vi "get Error Code.vi"(8 "error in":errorcluster, 10 "errorNum":u32, 11 "cycloneHandle":u32) -> (0 "error out":errorcluster, 3 "function return":i32)   [LabVIEW 2021, in "CycloneControlSDK.lvlib"]
doc: "extern \"C\" int32_t _cdecl getErrorCode(uint32_t cycloneHandle, uint32_t errorNum);"
uses:
  CycloneControlSDK.lvlib
  CycloneControlSDK_64.dll
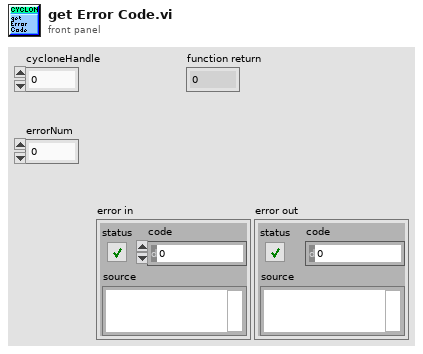
[diagram p1: front panel]
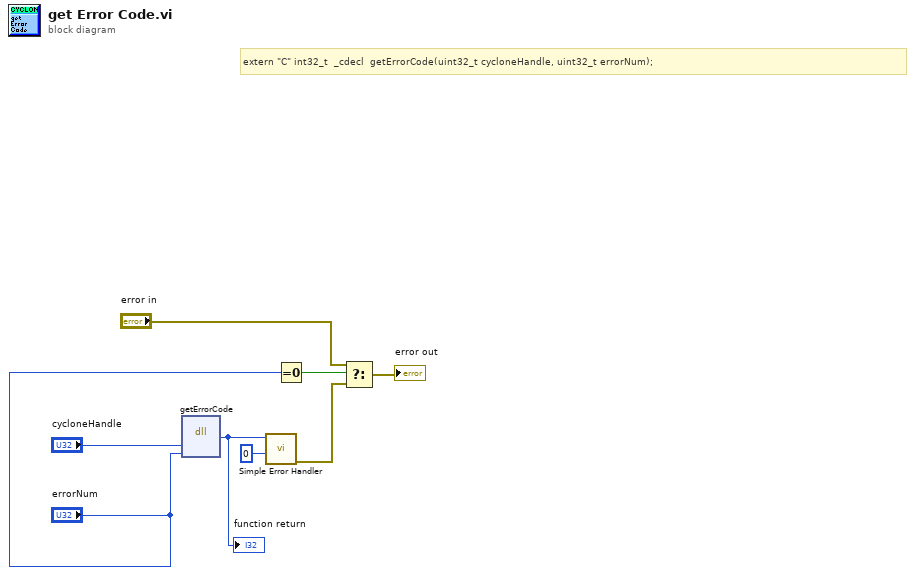
[diagram p0: block diagram]
diagram:
  # "extern \"C\" int32_t  _cdecl  getErrorCode(uint32_t cycloneHandle, uint32_t errorNum);"
  n1 = dll-call lib="C:/PEMicro/cyclone/cycloneControl/controlsdk/examples/labview2018/user.lib/CycloneControlSDK/CycloneControlSDK_64.dll" fn="getErrorCode"("cycloneHandle"="cycloneHandle", "errorNum"="errorNum") -> ("return type"=w6:i32)  [unwired: 5 in, 2 out]
  "function return" <- w6
  n2 = call <vilib>:"Simple Error Handler.vi"("error code (no error:0)"=w6, "type of dialog (OK msg:1)"=0) -> ("error out"=w4:errorcluster)  [unwired: 3 in, 4 out]
  n3 = Equal To 0?(x="errorNum") -> (x = 0?=w3:bool)
  n4 = Select(t="error in", s=w3, f=w4) -> (s? t:f=→"error out":errorcluster)
